vi "CloseSF.vi"(0 "error out":errorcluster, 2 "connection ID":refnum<k5>) -> ()   [LabVIEW 2009]
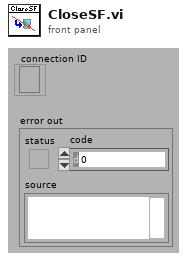
[diagram p1: front panel]
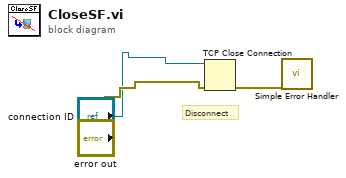
[diagram p0: block diagram]
diagram:
  # "Disconnect"
  n1 = TCP Close Connection(connection ID="connection ID", error in (no error)="error out") -> (error out=w1:errorcluster)  [unwired: 1 in, 1 out]
  n2 = call <vilib>:"Simple Error Handler.vi"("error in (no error)"=w1) -> ()  [unwired: 1 in, 8 out]
